vi "Get System Definition Schema Path.vi"() -> (3 "system definition schema path":string)   [LabVIEW 2017, in "Import Export.lvlib"]
uses:
  Import Export.lvlib
  NationalInstruments.VeriStand.SystemStorage
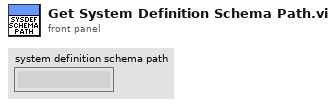
[diagram p1: front panel]
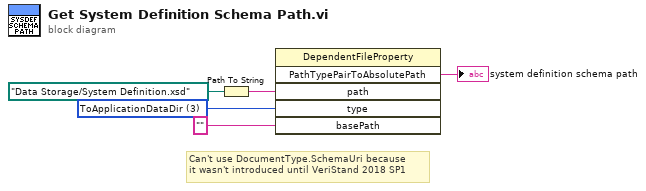
[diagram p0: block diagram]
diagram:
  w2 = 3 items=["Absolute", "Relative", "ToCommonDocDir", "ToApplicationDataDir"] ("type")
  # "Can't use DocumentType.SchemaUri because\nit wasn't introduced until VeriStand 2018 SP1"
  n1 = Path To String(path=path "Data Storage/System Definition.xsd") -> (string=w5:string)
  n2 = invoke class="DependentFileProperty" method="PathTypePairToAbsolutePath"("path"=w5, "type"=w2, "basePath"="") -> ("PathTypePairToAbsolutePath"=→"system definition schema path":string)  [unwired: 3 in, 5 out]
